vi "getchildren.vi"(3 "error in (no error)":errorcluster, 4 "Parent Tag":string, 5 "Tree Reference In":refnum<vi>) -> (0 "error out":errorcluster, 1 "Children Tags":string[](array[string]), 2 "Tree Reference Out":refnum<vi>)   [LabVIEW 2020]
doc: "This VI takes a tree control reference and a parent tag and returns an array of the children tags.\n\nYou can use this example as a subVI.\n\n1. Create a top level VI that contains tree control with at least one parent item that contains one or more child items.\n2. Place the GetChildren VI (this VI) on the block diagram of the top level VI.\n3. Create a reference to the tree by right-clicking the tree control and selecting <b>Create»Reference</b>.\n4. Wire the reference to the <b>Tree Reference In</b> input of the GetChildren VI.\n5. Place a string control on the front panel and type the parent item in the tree control whose children you want to return and wire the control to the <b>Parent Tag</b> input of the GetChildren VI. \n6. Create an indicator from the <b>Children Tags</b> output of the GetChildren VI.\n\nRun the VI and observe that this subVI returns all of the child items of the parent item in the tree that you referenced."
panel:
  # "Select Help»Show Context Help and move the cursor \nover the VI icon to display help for this VI."
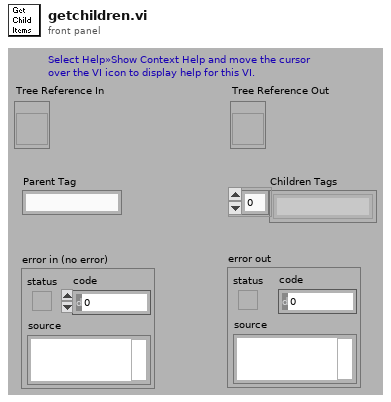
[diagram p1: front panel]
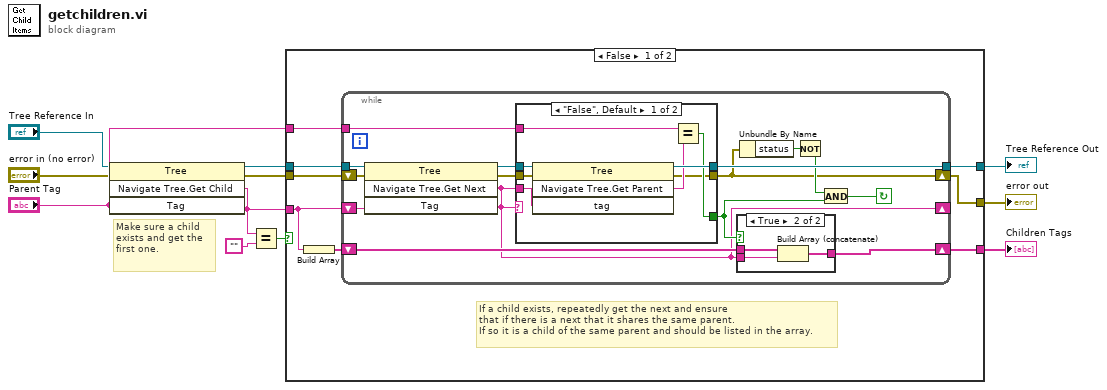
[diagram p0: block diagram]
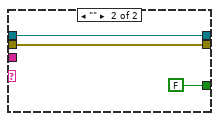
[diagram p2: hidden frame]
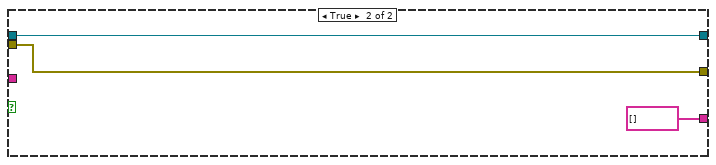
[diagram p4: hidden frame]
diagram:
  # "Make sure a child exists and get the first one."
  n1 = invoke class="Tree" method="Navigate Tree.Get Child"(reference="Tree Reference In", error in="error in (no error)", "Tag"="Parent Tag") -> (reference out=w9:refnum<vi>, error out=w7:errorcluster, "Navigate Tree:Get Child"=w5:string)  [unwired: 1 in, 1 out]
  n2 = Equal?(x=w5, y="") -> (x = y?=w4:bool)
  n3 = case shown="False" w4 {
    tunnel: "Parent Tag" -> [w19 _]
    tunnel: w5 -> [w18 _]
    tunnel: [w16 string[] []] -> w10
    tunnel: w9 -> [w15 w51]
    tunnel: [w14 w51] -> w1
    tunnel: w7 -> [w13 w52]
    tunnel: [w12 w52] -> w6
    frame False {
      # "If a child exists, repeatedly get the next and ensure \nthat if there is a next that it shares the same parent.\nIf so it is a child of the same parent and should be listed in the array."
      n4 = Build Array(w18) -> (w17:string[])
      n5 = while {
        tunnel: w15 -> [w34]
        tunnel: [w29] -> w14
        shift-right: [w32] -> w16
        shift-left: w17 -> [w33]
        shift-right: [w20] -> _
        shift-left: w18 -> [w31]
        tunnel: w19 -> [w28]
        shift-right: [w21] -> w12
        shift-left: w13 -> [w23]
        stop <- w26 continue-if-true
        n6 = invoke class="Tree" method="Navigate Tree.Get Next"(reference=w34, error in=w23, "Tag"=w31) -> (reference out=w30:refnum<vi>, error out=w22:errorcluster, "Navigate Tree:Get Next Item"=w20:string)  [unwired: 1 in, 1 out]
        n7 = case shown="\"False\", Default" w20 {
          tunnel: w30 -> [w42 w45]
          tunnel: [w41 w45] -> w29
          tunnel: w28 -> [w40 _]
          tunnel: w20 -> [w38 _]
          tunnel: [w37 FALSE] -> w27
          tunnel: w22 -> [w36 w44]
          tunnel: [w35 w44] -> w21
          frame "False", Default {
            n8 = invoke class="Tree" method="Navigate Tree.Get Parent"(reference=w42, error in=w36, "tag"=w38) -> (reference out=w41:refnum<vi>, error out=w35:errorcluster, "Navigate Tree:Get Parent"=w39:string)  [unwired: 1 in, 1 out]
            n9 = Equal?(x=w40, y=w39) -> (x = y?=w37:bool)
          }
          frame "" {
          }
        }
        n10 = case shown="True" w27 {
          tunnel: w33 -> [w46 w49]
          tunnel: [w46 w48] -> w32
          tunnel: w20 -> [_ w47]
          frame False {
          }
          frame True {
            n11 = Build Array (concatenate)(w49, w47) -> (w48:string[])
          }
        }
        n12 = Unbundle By Name(w21) -> ("status"=w25:bool)
        n13 = Not(x=w25) -> (.not. x?=w24:bool)
        n14 = And(x=w24, y=w27) -> (x .and. y?=w26:bool)
      }
    }
    frame True {
    }
  }
  "Children Tags" <- w10
  "error out" <- w6
  "Tree Reference Out" <- w1
